vi "MotorTest.vi"() -> ()   [LabVIEW 2018]
panel:
  in  "角度":dbl
  out "反馈位置":i32[](array[numeric])
  out "err out":u16[](array[numeric])
  out "绝对运动":i32
  in  "绝对运动":bool
  in  "脉冲":i32
  out "反向":i32
  out "正向":i32
  out "位置":i32
  in  "关机":bool
  in  "停止":bool
  in  "反向":bool
  in  "正向":bool
  out "运动":i32
  out "设置加速度减速度":i32
  out "限位使能":i32
  out "电机使能":i32
  out "编码器使能":i32
  out "方向设置成功":i32
  out "当前位置":i32[](array[numeric])
  out "逻辑位置返回":i32
  out "逻辑位置":i32[](array[numeric])
  out "型号":u32 format="%x"
  out "打开状态":u32
  out "网卡序号":i32[](array[numeric])
  out "网卡名":string[](array[string])
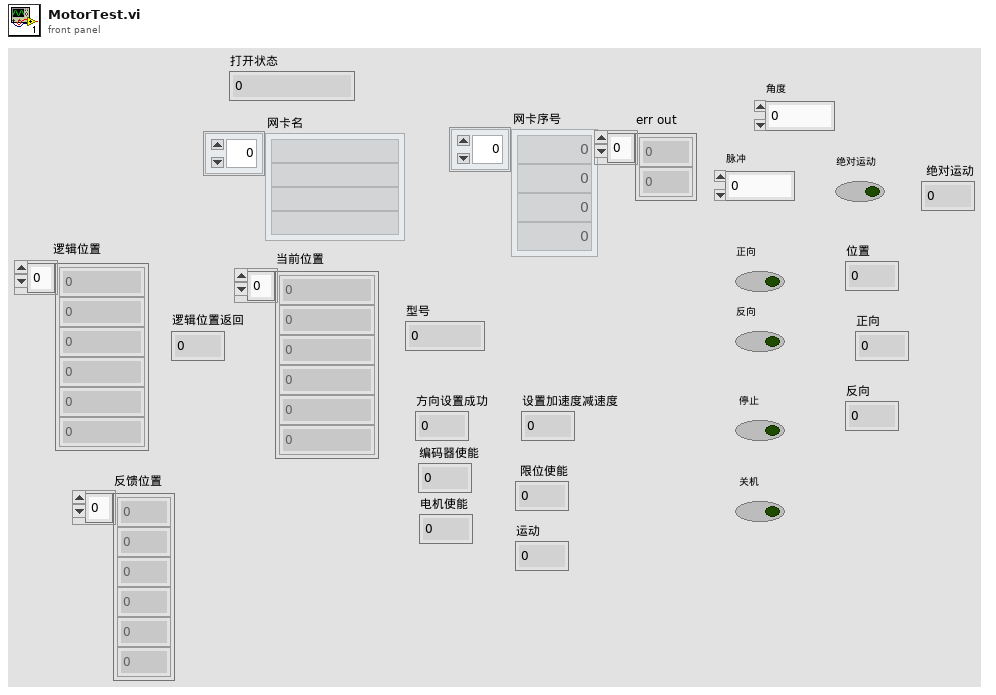
[diagram p1: front panel]
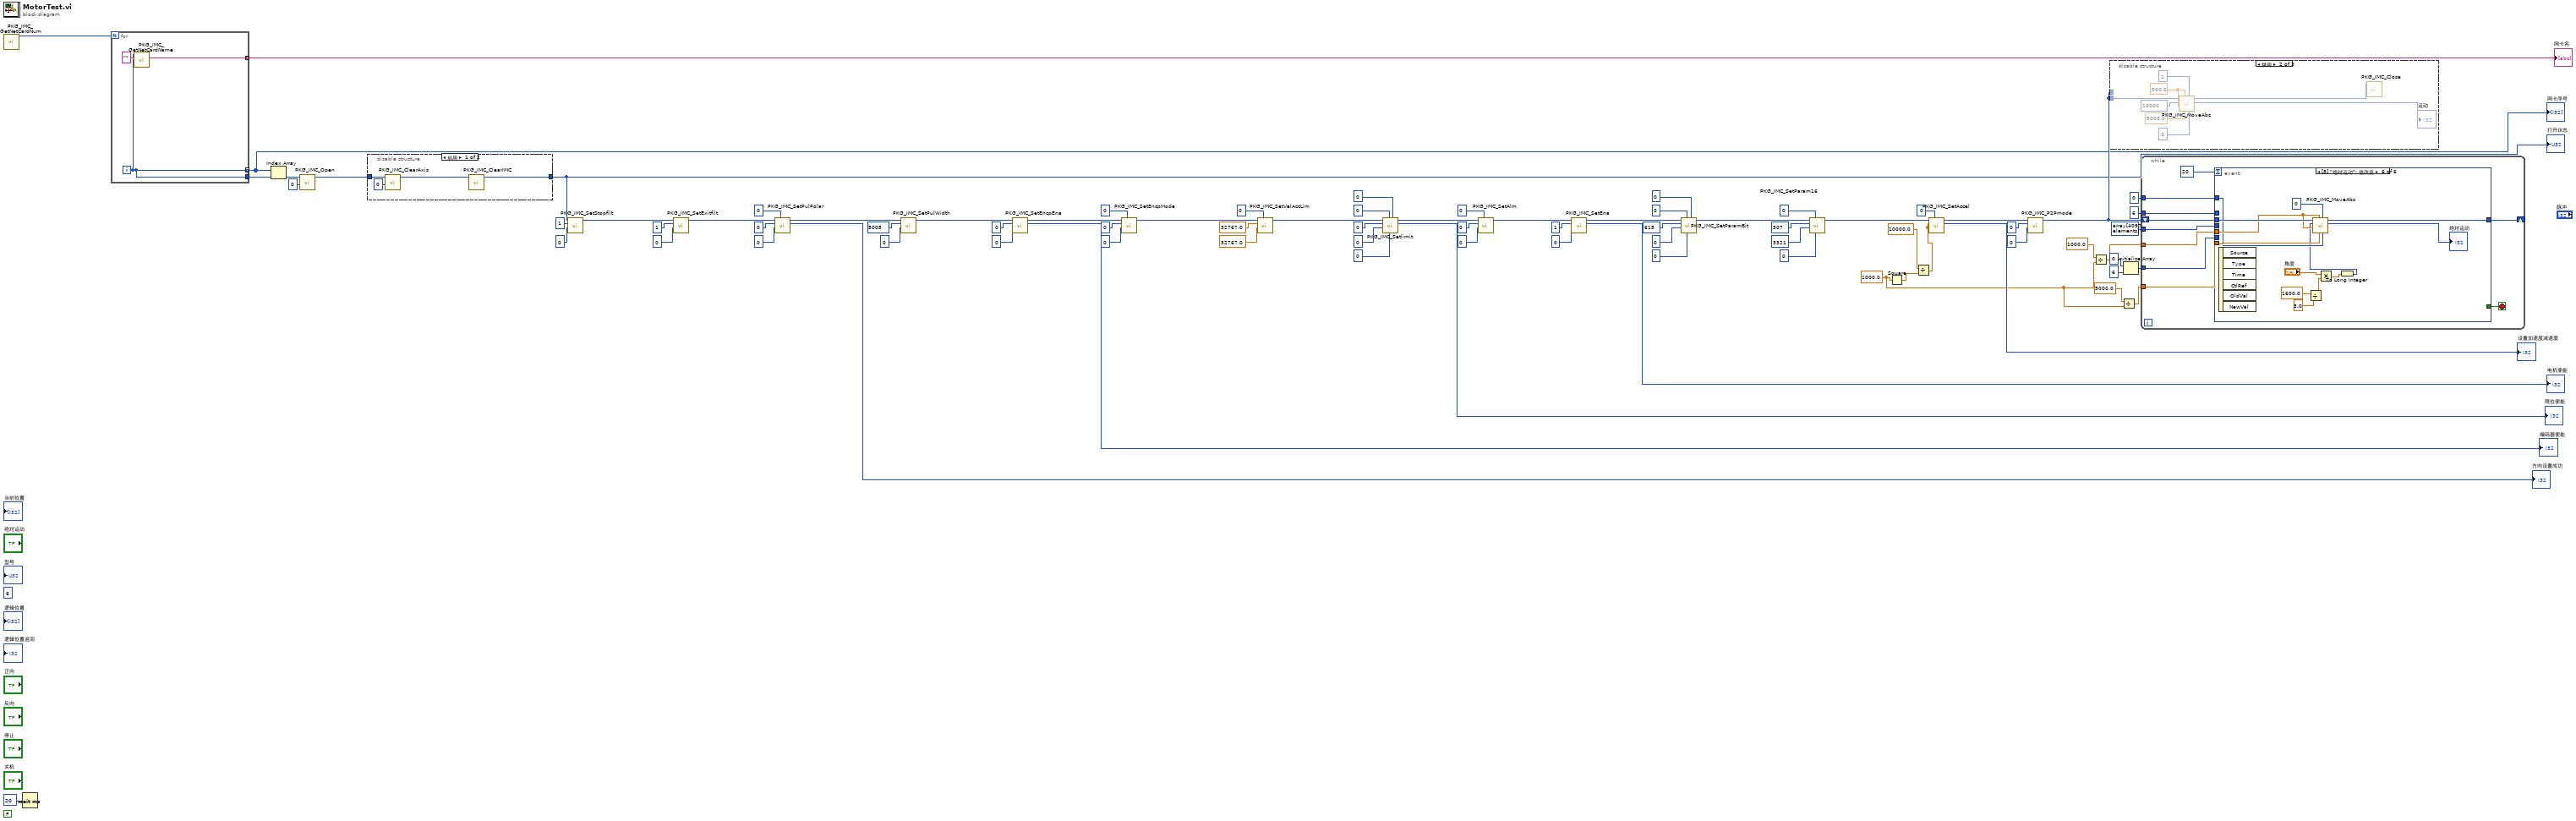
[diagram p0: block diagram]
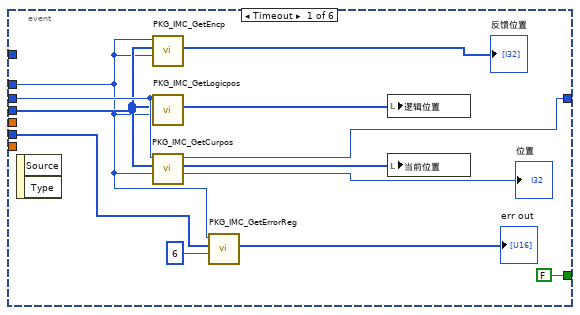
[diagram p2: hidden frame]
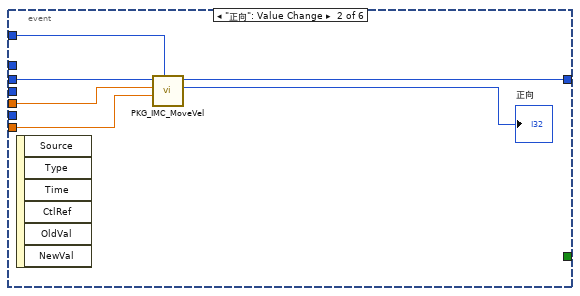
[diagram p3: hidden frame]
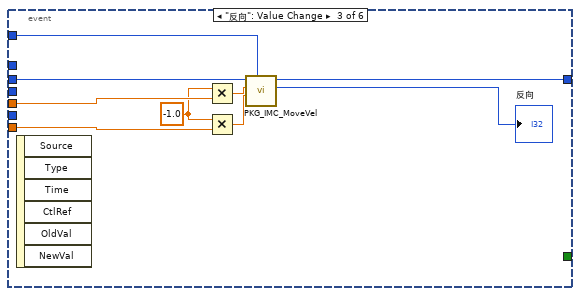
[diagram p4: hidden frame]
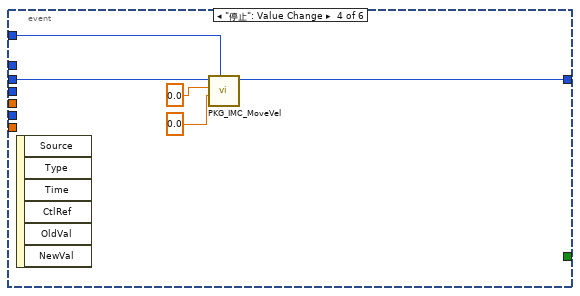
[diagram p5: hidden frame]
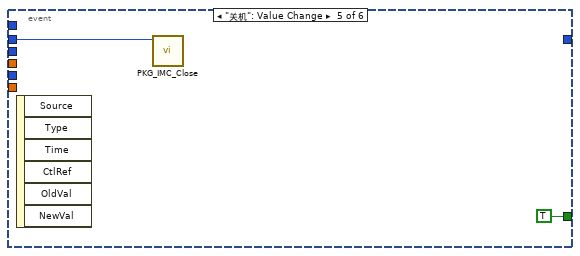
[diagram p6: hidden frame]
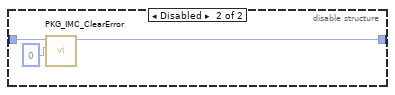
[diagram p7: hidden frame]
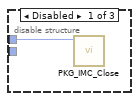
[diagram p8: hidden frame]
diagram:
  w4 = 1000.0
  (unwired) FALSE
  (unwired) 6 ("axisnum")
  n1 = call "PKG_IMC_GetNetCardNum.vi"() -> ("function return"=w81:i32)  [unwired: 11 in]
  n2 = Wait (ms)(milliseconds to wait=u32 20 ("等待时间（毫秒）")) -> ()  [unwired: 1 out]
  n3 = for {
    N: w81 -> [_]
    tunnel: [w83] -> w80 mode=indexing
    tunnel: [w82] -> w2 mode=indexing
    tunnel: [w82] -> w1
    i -> [w82]
    n4 = call "PKG_IMC_GetNetCardName.vi"("name"="", "index"=w82) -> ("name out"=w83:string)  [unwired: 8 in, 1 out]
  }
  "网卡名" <- w80
  "网卡序号" <- w2
  n5 = Index Array(array=w2, index=w1) -> (element=w79:i32)
  n6 = call "PKG_IMC_Open.vi"("imcid"=0, "netcardsel"=w79) -> ("function return"=w77:u32)  [unwired: 9 in]
  n7 = disable-structure shown="启用" {
    disable-tunnel: w77 -> [w88 w91]
    disable-tunnel: [w85 w89] -> w45
    frame Enabled {
      n8 = call "PKG_IMC_ClearAxis.vi"("axis"=0, "handle"=w88) -> ("handle out"=w86:u32)  [unwired: 8 in, 1 out]
      n9 = call "PKG_IMC_ClearIMC.vi"("handle"=w86) -> ("handle out"=w85:u32)  [unwired: 9 in, 1 out]
    }
    frame Disabled {
      n10 = call "PKG_IMC_ClearError.vi"("axis"=0, "Handle"=w91) -> ("Handle out"=w89:u32)  [unwired: 8 in, 1 out]
    }
  }
  "打开状态" <- w45
  n11 = call "PKG_IMC_SetStopfilt.vi"("axis"=0, "stop"=1, "handle"=w45) -> ("handle out"=w42:u32)  [unwired: 7 in, 1 out]
  n12 = call "PKG_IMC_SetExitfilt.vi"("axis"=0, "exit"=1, "handle"=w42) -> ("handle out"=w39:u32)  [unwired: 7 in, 1 out]
  n13 = call "PKG_IMC_SetPulPolar.vi"("axis"=0, "dir"=0, "pul"=0, "handle"=w39) -> ("function return"=→"方向设置成功":i32, "handle out"=w52:u32)  [unwired: 6 in]
  n14 = call "PKG_IMC_SetPulWidth.vi"("axis"=0, "ns"=u32 5005, "handle"=w52) -> ("handle out"=w51:u32)  [unwired: 7 in, 1 out]
  n15 = call "PKG_IMC_SetEncpEna.vi"("axis"=0, "ena"=0, "handle"=w51) -> ("function return"=→"编码器使能":i32, "handle out"=w38:u32)  [unwired: 7 in]
  n16 = call "PKG_IMC_SetEncpMode.vi"("axis"=0, "dir"=0, "mode"=0, "handle"=w38) -> ("handle out"=w34:u32)  [unwired: 6 in, 1 out]
  n17 = call "PKG_IMC_SetVelAccLim.vi"("axis"=0, "acclim"=32767.0, "vellim"=32767.0, "handle"=w34) -> ("handle out"=w30:u32)  [unwired: 6 in, 1 out]
  n18 = call "PKG_IMC_Setlimit.vi"("axis"=0, "nlimPolar"=0, "nlimEna"=0, "plimPolar"=0, "plimEna"=0, "handle"=w30) -> ("function return"=→"限位使能":i32, "handle out"=w29:u32)  [unwired: 4 in]
  n19 = call "PKG_IMC_SetAlm.vi"("axis"=0, "polar"=0, "ena"=0, "handle"=w29) -> ("handle out"=w23:u32)  [unwired: 6 in, 1 out]
  n20 = call "PKG_IMC_SetEna.vi"("axis"=0, "ena"=1, "handle"=w23) -> ("function return"=→"电机使能":i32, "handle out"=w22:u32)  [unwired: 7 in]
  n21 = call "PKG_IMC_SetParamBit.vi"("fifo"=0, "axis"=0, "val"=i16 0, "bit"=i16 0, "paramloc"=i16 615, "Handle"=w22) -> ("Handle out"=w16:u32)  [unwired: 4 in, 1 out]
  n22 = call "PKG_IMC_SetParam16.vi"("fifo"=0, "axis"=0, "data"=i16 3321, "paramloc"=i16 307, "Handle"=w16) -> ("Handle out"=w11:u32)  [unwired: 5 in, 1 out]
  n23 = Square(x=w4) -> (x^2=w9:dbl)
  n24 = Divide(x=10000.0 ("accel"), y=w9) -> (x/y=w8:dbl)
  n25 = call "PKG_IMC_SetAccel.vi"("axis"=0, "decel"=w8, "accel"=w8, "handle"=w11) -> ("function return"=→"设置加速度减速度":i32, "handle out"=w56:u32)  [unwired: 6 in]
  n26 = call "PKG_IMC_P2Pmode.vi"("axis"=0, "mode"=0, "handle"=w56) -> ("handle out"=w53:u32)  [unwired: 7 in, 1 out]
  n27 = Divide(x=1000.0, y=w4) -> (x/y=w6:dbl)
  n28 = disable-structure shown="禁用" {
    disable-tunnel: w53 -> [_ w94 _]
    disable-tunnel: w53 -> [w92 _ _]
    frame Disabled {
      n29 = call "PKG_IMC_Close.vi"("Handle"=w92) -> ()  [unwired: 9 in, 2 out]
    }
    frame Disabled {
      w96 = 500.0 ("startvel")
      n30 = call "PKG_IMC_MoveAbs.vi"("axis"=0, "wait"=1, "tgvel"=5000.0, "endvel"=w96, "startvel"=w96, "pos"=10000, "handle"=w94) -> ("function return"=→"运动":i32, "handle out"=w93:u32)  [unwired: 3 in]
      n31 = call "PKG_IMC_Close.vi"("Handle"=w93) -> ()  [unwired: 9 in, 2 out]
    }
    frame Enabled {
    }
  }
  n32 = Divide(x=5000.0, y=w4) -> (x/y=w3:dbl)
  n33 = Initialize Array(u8 0 ("元素"), 6 ("维数大小")) -> (w46:u8[])
  n34 = while {
    shift-right: [w107] -> _
    shift-left: w53 -> [w108]
    tunnel: i32[] array[4097 elements] ("pos") -> [w106]
    tunnel: 0 ("axisnum") -> [w105]
    tunnel: w6 -> [w104]
    tunnel: w3 -> [w103]
    tunnel: 6 ("axisnum") -> [w102]
    tunnel: w46 -> [w101]
    stop <- w110 stop-if-true
    n35 = event shown="[5] \"绝对运动\": 值改变" {
      selector: _ -> [_ _ _ _ _ _]
      dyn-events: _ -> [_ _ _ _ _ _]
      timeout: 20 -> [_ _ _ _ _ _]
      tunnel: [FALSE _ _ _ TRUE _] -> w110
      tunnel: w108 -> [w117 w128 w137 w141 w144 w157]
      tunnel: [w121 w127 w130 w140 _ w156] -> w107
      tunnel: w106 -> [w113 _ _ _ _ _]
      tunnel: w105 -> [_ w124 w131 w142 _ w153]
      tunnel: w104 -> [_ w126 w136 _ _ w155]
      tunnel: w103 -> [_ w125 w133 _ _ w154]
      tunnel: w102 -> [w111 _ _ _ _ _]
      tunnel: w101 -> [w116 _ _ _ _ _]
      event Timeout {
        n36 = event-data() -> ()  [unwired: 1 in, 2 out]
        n37 = call "PKG_IMC_GetEncp.vi"("axisnum"=w111, "pos"=w113, "Handle"=w111) -> ("pos out"=→"反馈位置":i32[])  [unwired: 6 in, 2 out]
        n38 = call "PKG_IMC_GetLogicpos.vi"("axisnum"=w111, "pos"=w113, "Handle"=w117) -> ("pos out"=w118:i32[])  [unwired: 6 in, 2 out]
        n39 = call "PKG_IMC_GetCurpos.vi"("axisnum"=w111, "pos"=w113, "Handle"=w117) -> ("function return"=→"位置":i32, "pos out"=w120:i32[], "Handle out"=w121:u32)  [unwired: 6 in]
        n40 = call "PKG_IMC_GetErrorReg.vi"("axisnum"=6, "err"=w116, "Handle"=w111) -> ("err out"=→"err out":u16[])  [unwired: 6 in, 2 out]
        n41 = local write "逻辑位置"(w118) -> ()
        n42 = local write "当前位置"(w120) -> ()
      }
      event "正向": Value Change {
        n43 = event-data() -> ()  [unwired: 1 in, 6 out]
        n44 = call "PKG_IMC_MoveVel.vi"("axis"=w124, "tgvel"=w125, "startvel"=w126, "handle"=w128) -> ("function return"=→"正向":i32, "handle out"=w127:u32)  [unwired: 6 in]
      }
      event "反向": Value Change {
        w134 = -1.0 ("x")
        n45 = event-data() -> ()  [unwired: 1 in, 6 out]
        n46 = Multiply(x=w134, y=w136) -> (x*y=w135:dbl)
        n47 = Multiply(x=w134, y=w133) -> (x*y=w132:dbl)
        n48 = call "PKG_IMC_MoveVel.vi"("axis"=w131, "tgvel"=w132, "startvel"=w135, "handle"=w137) -> ("function return"=→"反向":i32, "handle out"=w130:u32)  [unwired: 6 in]
      }
      event "停止": Value Change {
        n49 = event-data() -> ()  [unwired: 1 in, 6 out]
        n50 = call "PKG_IMC_MoveVel.vi"("axis"=w142, "tgvel"=0.0, "startvel"=0.0, "handle"=w141) -> ("handle out"=w140:u32)  [unwired: 6 in, 1 out]
      }
      event "关机": Value Change {
        n51 = event-data() -> ()  [unwired: 1 in, 6 out]
        n52 = call "PKG_IMC_Close.vi"("Handle"=w144) -> ()  [unwired: 9 in, 2 out]
      }
      event "绝对运动": Value Change {
        n53 = event-data() -> ()  [unwired: 1 in, 6 out]
        n54 = Divide(x=1600.0, y=3.0) -> (x/y=w147:dbl)
        n55 = Multiply(x="角度", y=w147) -> (x*y=w146:dbl)
        n56 = To Long Integer(number=w146) -> (32bit integer=w145:i32)
        n57 = call "PKG_IMC_MoveAbs.vi"("axis"=w153, "wait"=0, "tgvel"=w154, "endvel"=w155, "startvel"=w155, "pos"=w145, "handle"=w157) -> ("function return"=→"绝对运动":i32, "handle out"=w156:u32)  [unwired: 3 in]
      }
    }
  }
